vi "init.vi"(8 "error in (no error)":errorcluster, 11 "Input":string="34,45,89") -> (0 "error out":errorcluster, 3 "Output":string)   [LabVIEW 2014]
uses:
  <userlib>/Nanonis Prog Interface V5/Nanonis Prog Interface.lvlib
panel:
  in  "Bias (V)":sgl=-1.0 format="%_5p"
  in  "Z Controller setpoint":sgl=2.5e-11 format="%#_6p"
  in  "Speed (m/s)":cluster{"Forward":sgl, "Backward":sgl}={"Forward"=8e-08, "Backward"=1.6e-07} caption="Speed (m/s) (NaN=no change)" {"Backward" format="%.2p"; "Forward" format="%.2p"}
  # "."
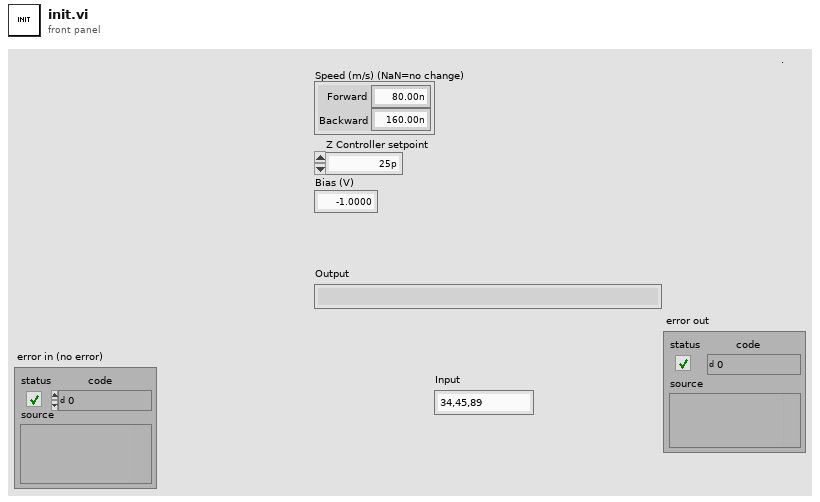
[diagram p1: front panel]
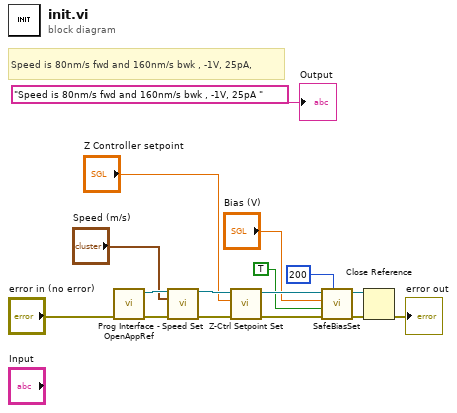
[diagram p0: block diagram]
diagram:
  # "Speed is 80nm/s fwd and 160nm/s bwk , -1V, 25pA,"
  n1 = call <userlib>:"Prog Interface - OpenAppRef.vi"("Error in (no error)"="error in (no error)") -> ("Error out"=w13:errorcluster, "Application reference"=w14:refnum<vi>)  [unwired: 5 in]
  n2 = call <userlib>:"Speed Set.vi"("Application ref in"=w14, "Speed (m/s)"="Speed (m/s)", "error in (no error)"=w13) -> ("Application ref out"=w8:refnum<vi>, "error out"=w12:errorcluster)  [unwired: 11 in]
  n3 = call <userlib>:"Z-Ctrl Setpoint Set.vi"("error in (no error)"=w12, "Z Controller setpoint"="Z Controller setpoint", "Application ref in"=w8) -> ("error out"=w11:errorcluster, "Application ref out"=w7:refnum<vi>)  [unwired: 7 in]
  n4 = call "SafeBiasSet.vi"("Application ref in"=w7, "Bias (V)"="Bias (V)", "Ramp"=TRUE, "error in (no error)"=w11, "milliseconds to wait"=u32 200) -> ("Application ref out"=w10:refnum<vi>, "Error out"=w9:errorcluster)  [unwired: 4 in]
  n5 = Close Reference(reference=w10, error in (no error)=w9) -> (error out=→"error out":errorcluster)
  "Output" <- "Speed is 80nm/s fwd and 160nm/s bwk , -1V, 25pA " ("Output")
